vi "machine_State.vi"() -> ()   [LabVIEW 2020]
uses:
  <vilib>/ErrorRing/Error Ring.xnode
panel:
  out "Array 2":bool[](array[boolean])
  out "Array":dbl[](array[slide]) scale=0.0..100.0
  in  "Alarmas":dbl(slide) scale=0.0..100.0
  in  "stop":bool
  out "Estado Actual":string
  in  "Data_Analisis.Direccion":path
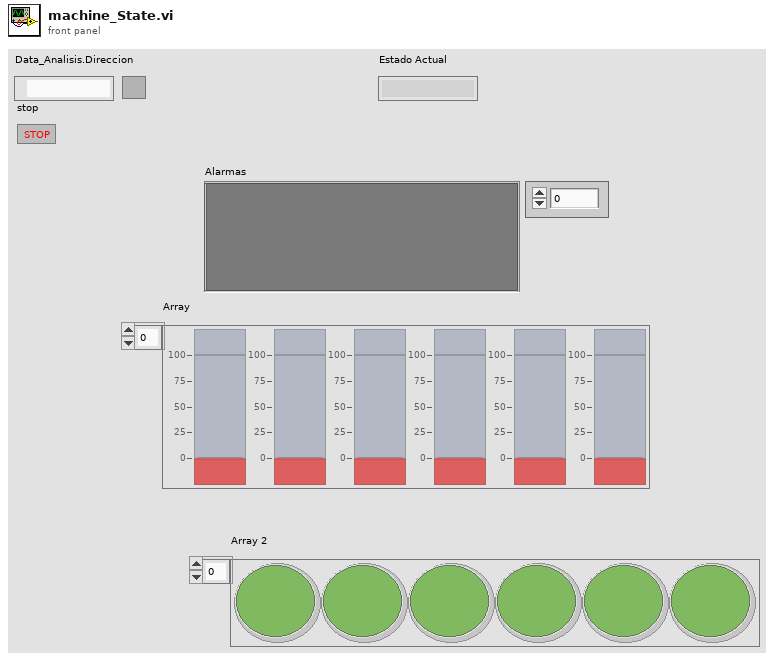
[diagram p1: front panel]
types:
  T1 = cluster{"Hardaware":cluster{"Data Value":dbl[]}, "Data_Analisis":cluster{"Formato":string, "Nombre del Fichero":string, "Direccion":path, "refnum out":refnum<file>}, "N values":cluster{"N max":i32, "L_Min":dbl, "L_Max":dbl}, "Warnings":cluster{"Alarmas":bool[]}}
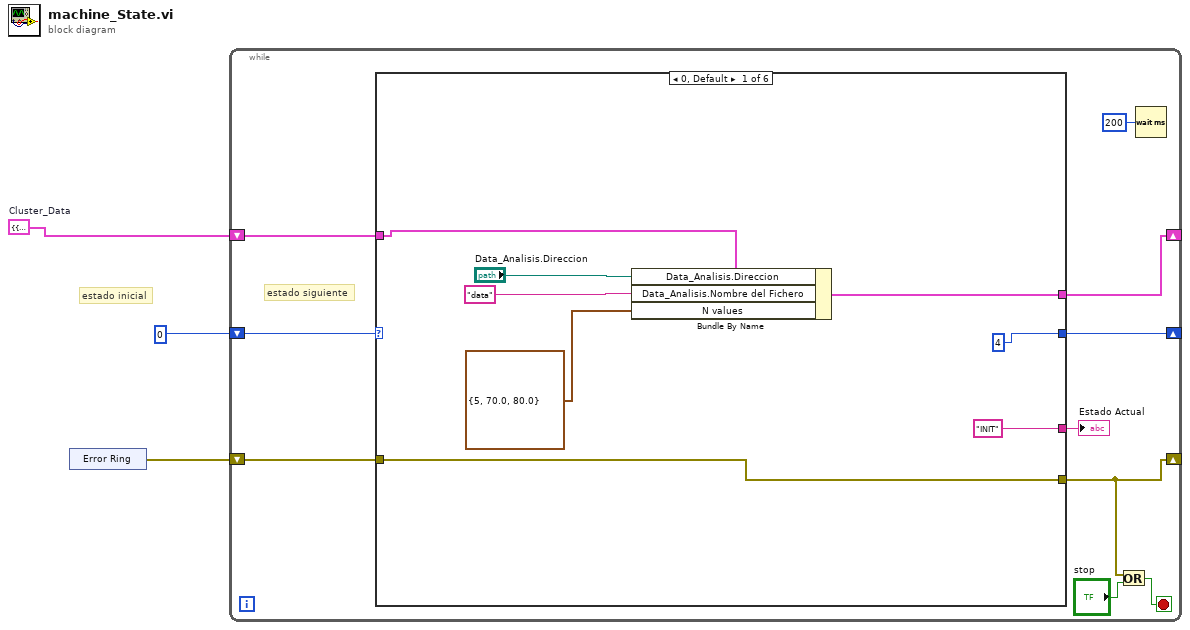
[diagram p0: block diagram]
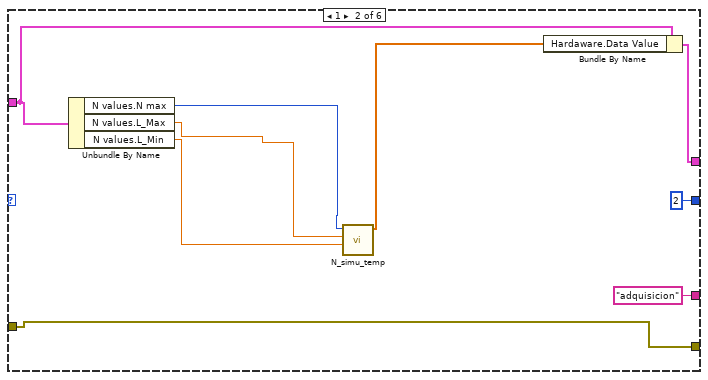
[diagram p2: hidden frame]
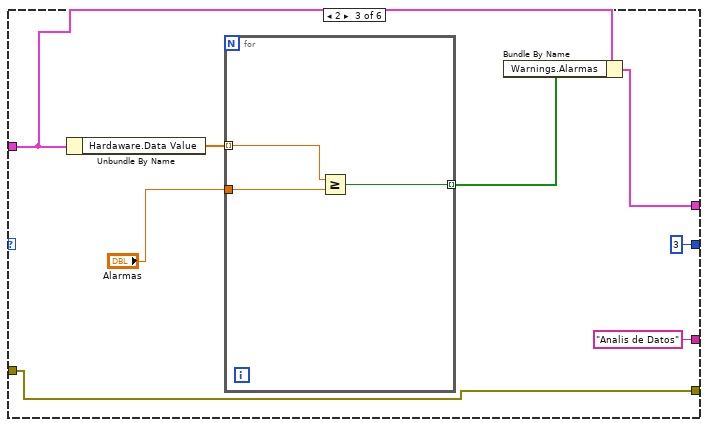
[diagram p3: hidden frame]
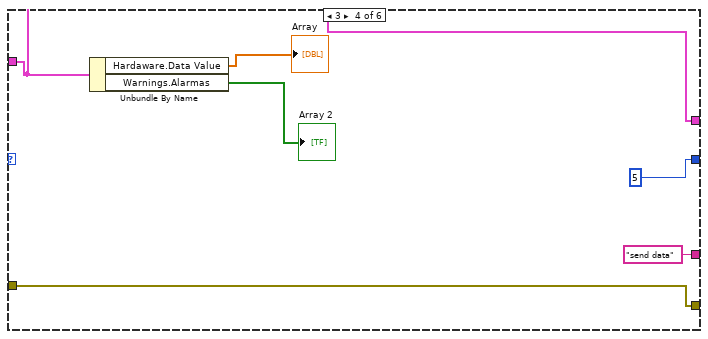
[diagram p4: hidden frame]
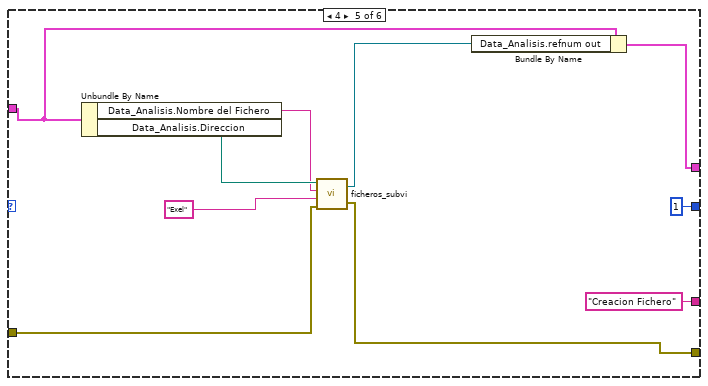
[diagram p5: hidden frame]
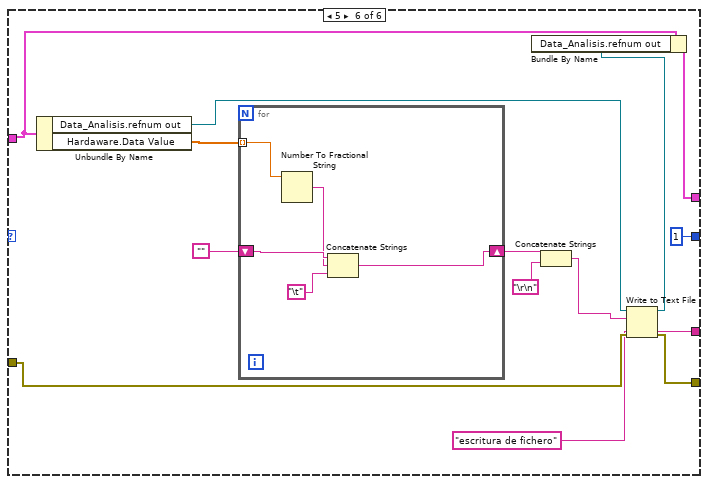
[diagram p6: hidden frame]
diagram:
  w2 = T1 {"Hardaware"={"Data Value"=[]}, "Data_Analisis"={"Formato"="", "Nombre del Fichero"="", "Direccion"=path "", "refnum out"=refnum}, "N values"={"N max"=0, "L_Min"=0.0, "L_Max"=0.0}, "Warnings"={"Alarmas"=[FALSE]}}  # Cluster_Data
  # "estado inicial"
  n1 = xnode "Error Ring"() -> ("error out"=w1:errorcluster)
  n2 = while {
    shift-right: [w11] -> _
    shift-left: w2 -> [w12]
    shift-right: [w9] -> _
    shift-left: 0 -> [w13]
    shift-right: [w5] -> _
    shift-left: w1 -> [w7]
    stop <- w4 stop-if-true
    # "estado siguiente"
    n3 = case shown="0, Default" w13 {
      tunnel: w12 -> [w21 w26 w35 w44 w52 w62]
      tunnel: [w17 w24 w33 w44 w50 w60] -> w11
      tunnel: [4 2 3 5 1 1] -> w9
      tunnel: ["INIT" "adquisicion" "Analis de Datos" "send data" "Creacion Fichero" "escritura de fichero"] -> w8
      tunnel: [w14 w27 w36 w45 w53 w63] -> w5
      tunnel: w7 -> [w14 w27 w36 w45 w54 w64]
      frame 0, Default {
        n4 = Bundle By Name(cluster=w21, "Data_Analisis.Direccion"="Data_Analisis.Direccion", "Data_Analisis.Nombre del Fichero"="data", "N values"=cluster{i32, dbl, dbl} {5, 70.0, 80.0}) -> (w17:T1)
      }
      frame 1 {
        n5 = Unbundle By Name(w26) -> ("N values.N max"=w30:i32, "N values.L_Max"=w29:dbl, "N values.L_Min"=w28:dbl)
        n6 = call "N_simu_temp.vi"("Lmini"=w28, "L max"=w29, "N"=w30) -> ("Array"=w25:dbl[])  [unwired: 8 in]
        n7 = Bundle By Name(cluster=w26, "Hardaware.Data Value"=w25) -> (w24:T1)
      }
      frame 2 {
        n8 = Unbundle By Name(w35) -> ("Hardaware.Data Value"=w38:dbl[])
        n9 = for {
          tunnel: w38 -> [w41] mode=indexing
          tunnel: "Alarmas" -> [w40]
          tunnel: [w39] -> w34 mode=indexing
          n10 = Greater Or Equal?(x=w41, y=w40) -> (x >= y?=w39:bool)
        }
        n11 = Bundle By Name(cluster=w35, "Warnings.Alarmas"=w34) -> (w33:T1)
      }
      frame 3 {
        n12 = Unbundle By Name(w44) -> ("Hardaware.Data Value"=→"Array":dbl[], "Warnings.Alarmas"=→"Array 2":bool[])
      }
      frame 4 {
        n13 = Unbundle By Name(w52) -> ("Data_Analisis.Nombre del Fichero"=w56:string, "Data_Analisis.Direccion"=w57:path)
        n14 = call "ficheros_subvi.vi"("error in (no error)"=w54, "Formato"="Exel", "Nombre del Archivo"=w56, "Ruta de Almacenamiento"=w57) -> ("error out"=w53:errorcluster, "Byte Stream File out"=w51:refnum<file>)
        n15 = Bundle By Name(cluster=w52, "Data_Analisis.refnum out"=w51) -> (w50:T1)
      }
      frame 5 {
        n16 = Unbundle By Name(w62) -> ("Data_Analisis.refnum out"=w66:refnum<file>, "Hardaware.Data Value"=w70:dbl[])
        n17 = for {
          tunnel: w70 -> [w75] mode=indexing
          shift-right: [w71] -> w68
          shift-left: "" -> [w74]
          n18 = Number To Fractional String(number=w75) -> (F-format string=w73:string)  [unwired: 3 in]
          n19 = Concatenate Strings(w74, w73, "\t") -> (w71:string)
        }
        n20 = Concatenate Strings(w68, "\r\n") -> (w65:string)
        n21 = Write to Text File(file (use dialog)=w66, text=w65, error in=w64) -> (refnum out=w61:refnum<file>, error out=w63:errorcluster)  [unwired: 1 in, 1 out]
        n22 = Bundle By Name(cluster=w62, "Data_Analisis.refnum out"=w61) -> (w60:T1)
      }
    }
    "Estado Actual" <- w8
    n23 = Or(x=w5, y="stop") -> (x .or. y?=w4:bool)
    n24 = Wait (ms)(milliseconds to wait=u32 200) -> ()  [unwired: 1 out]
  }
